vi "ZRANGE.vi"(0 "refnum in":refnum<vi>, 1 "Key":string, 2 "Option":enum16{"None", "WITHSCORES"}(ring), 5 "Start":string, 7 "Stop":string, 11 "error in":errorcluster) -> (4 "refnum out":refnum<vi>, 6 "Data":T1, 15 "error out":errorcluster)   [LabVIEW 2020]
uses:
  SubVIs/Controls/redis-data.ctl
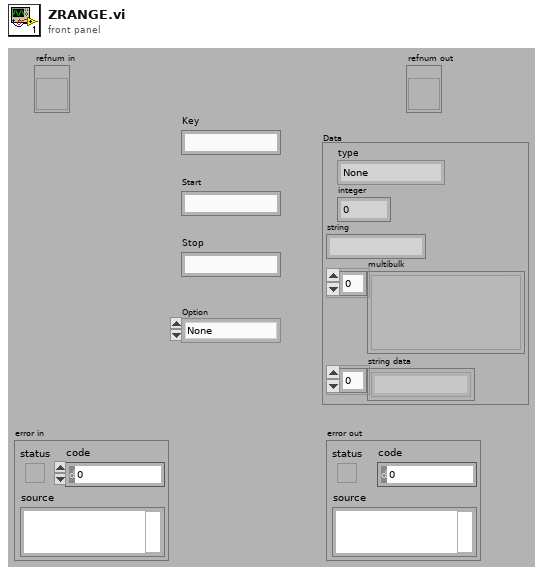
[diagram p1: front panel]
types:
  T1 = typedef "redis-data.ctl" = cluster{"type":enum16{"None", "Error", "Status", "Nil", "Integer", "String", "Multibulk"}, "integer":i64, "string":string, "multibulk":variant[], "string data":string[]}
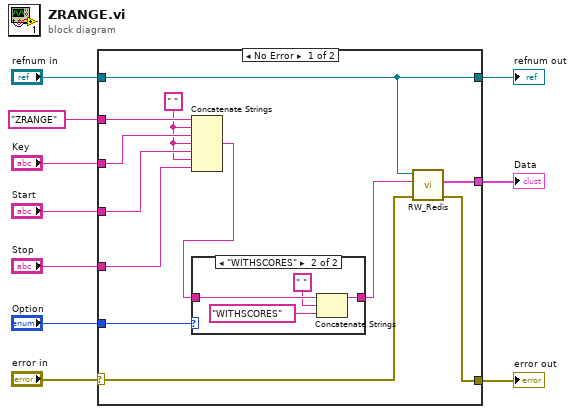
[diagram p0: block diagram]
diagram:
  n1 = case shown="No Error" "error in" {
    selector: "error in" -> [w21 w29]
    tunnel: "Key" -> [w18 _]
    tunnel: "ZRANGE" -> [w22 _]
    tunnel: "refnum in" -> [w17 w28]
    tunnel: [w20 w29] -> w8
    tunnel: [w19 _] -> w3
    tunnel: "Stop" -> [w12 _]
    tunnel: [w17 w28] -> w5
    tunnel: "Start" -> [w16 _]
    tunnel: "Option" -> [w15 _]
    frame No Error {
      w13 = " "
      n2 = Concatenate Strings(w22, w13, w18, w13, w16, w13, w12) -> (w11:string)
      n3 = case shown="\"WITHSCORES\"" w15 {
        tunnel: w11 -> [w23 w27]
        tunnel: [w23 w24] -> w14
        frame "None", Default {
        }
        frame "WITHSCORES" {
          n4 = Concatenate Strings(w27, " ", "WITHSCORES") -> (w24:string)
        }
      }
      n5 = call "RW_Redis.vi"("error in"=w21, "command"=w14, "refnum"=w17) -> ("error out"=w20:errorcluster, "Data"=w19:T1)  [unwired: 7 in]
    }
    frame Error {
    }
  }
  "error out" <- w8
  "Data" <- w3
  "refnum out" <- w5
